vi "Get SQL Formatted Value.vi"(8 "error in (no error)":errorcluster, 10 "Value":variant, 11 "String Value in":refnum<class "String Value.lvclass">) -> (0 "error out":errorcluster, 2 "SQL Formatted Value":string, 3 "String Value out":refnum<class "String Value.lvclass">)   [LabVIEW 2020, in "Composed Columns.lvlib" / "String Value.lvclass"]
uses:
  String Value.lvclass
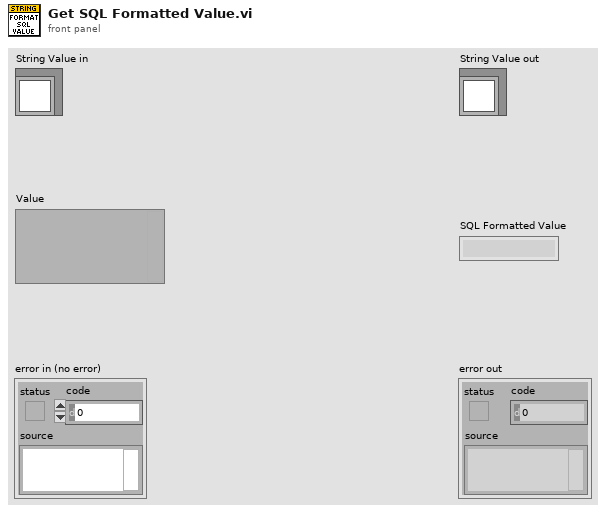
[diagram p1: front panel]
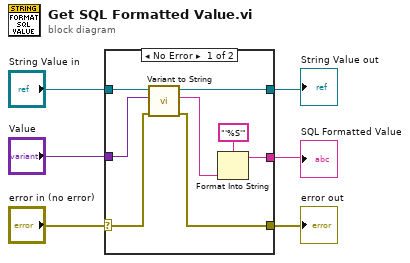
[diagram p0: block diagram]
diagram:
  n1 = case shown="No Error" "error in (no error)" {
    selector: "error in (no error)" -> [w11 w16]
    tunnel: [w10 w16] -> w2
    tunnel: [w13 w15] -> w5
    tunnel: "String Value in" -> [w14 w15]
    tunnel: "Value" -> [w12 _]
    tunnel: [w7 _] -> w3
    frame No Error {
      n2 = call-dynamic "Variant to String.vi"("error in (no error)"=w11, "Variant"=w12, "String Value in"=w14) -> ("error out"=w10:errorcluster, "String"=w8:string, "String Value out"=w13:refnum<class "String Value.lvclass">)  [unwired: 6 in]
      n3 = Format Into String(format string="'%S'", w8) -> (resulting string=w7:string)  [unwired: 2 in, 1 out]
    }
    frame Error {
    }
  }
  "error out" <- w2
  "String Value out" <- w5
  "SQL Formatted Value" <- w3
